vi "Read-Write File Paths setup.vi"(8 "error in":errorcluster, 11 "Function":T1) -> (0 "error out":errorcluster)   [LabVIEW 2020]
uses:
  Typedefs/Read Write Enum.ctl
  Typedefs/Which path.ctl
  Typedefs/File or Folder path or name.ctl
  Calibration/Globals/gl_Calibration globals.vi
  <vilib>/Utility/config.llb/Read Key (String).vi
  <vilib>/Utility/config.llb/NI_LVConfig.lvlib
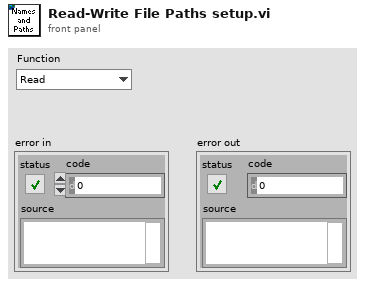
[diagram p1: front panel]
types:
  T1 = typedef "Read Write Enum.ctl" = enum16{"Read", "Write"}
  T2 = typedef "Which path.ctl" = enum16{"Configuration Files", "Calibration Files", "Images", "Setup.ini", "Loaded User profile.ini", "User's-Previous session.ini", "New user profile.ini", "Selected User profile.ini", "User profiles folder", "Power meter scaling.txt", "FOV Cal.ini", "Calibration.ini"}
  T3 = typedef "File or Folder path or name.ctl" = enum16{"Folder name", "Folder path", "File name", "File path & name"}
  T4 = typedef "NI_LVConfig.lvlib/Config Data RefNum.ctl" = refnum<k1>
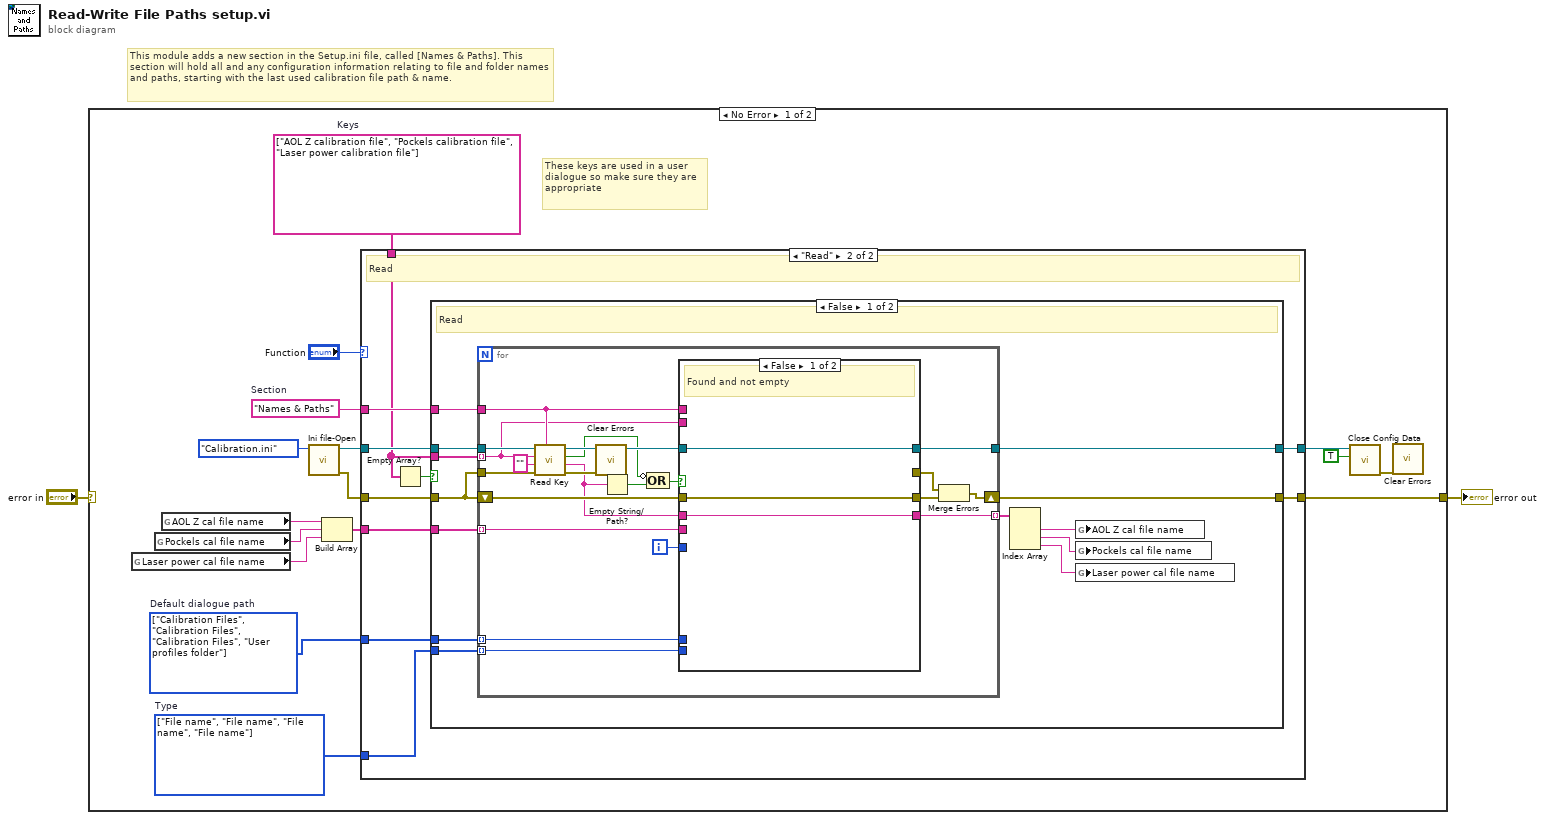
[diagram p0: block diagram]
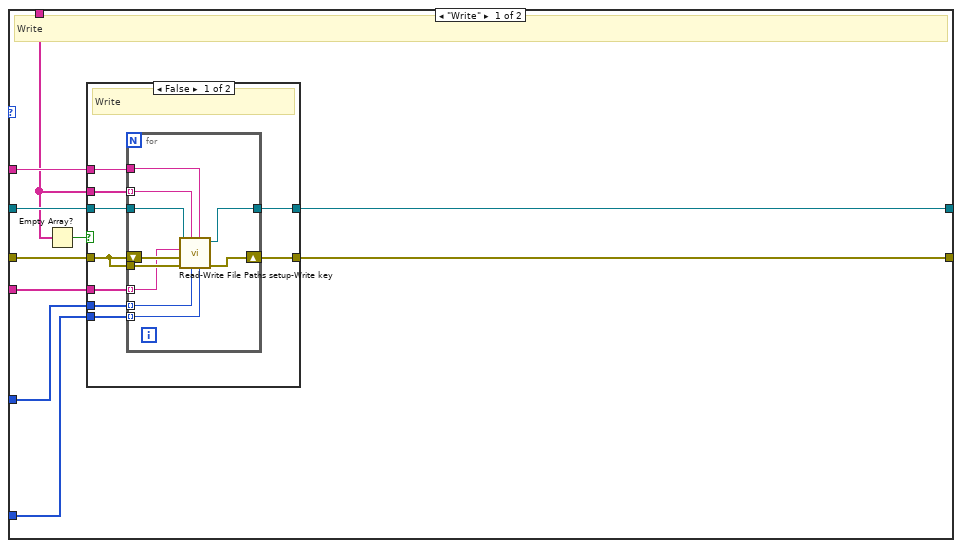
[diagram p2: hidden frame]
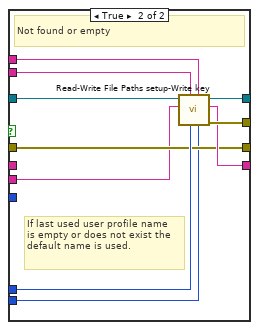
[diagram p4: hidden frame]
diagram:
  # "This module adds a new section in the Setup.ini file, called [Names & Paths]. This section will hold all and any configuration information relating to file and folder names and paths, starting with the last used calibration file path & name."
  n1 = case shown="No Error" "error in" {
    selector: "error in" -> [_ w109]
    tunnel: [w9 w109] -> w2
    frame No Error {
      w6 = T3[] [enum."File name", enum."File name", enum."File name", enum."File name"] items=["Folder name", "Folder path", "File name", "File path & name"]  # Type
      w7 = T2[] [enum."Calibration Files", enum."Calibration Files", enum."Calibration Files", enum."User profiles folder"] items=["Configuration Files", "Calibration Files", "Images", "Setup.ini", "Loaded User profile.ini", "User's-Previous session.ini", "New user profile.ini", "Selected User profile.ini", "User profiles folder", "Power meter scaling.txt", "FOV Cal.ini", "Calibration.ini"]  # Default dialogue path
      w11 = string[] ["AOL Z calibration file", "Pockels calibration file", "Laser power calibration file"]  # Keys
      w18 = "Names & Paths"  # Section
      # "These keys are used in a user dialogue so make sure they are appropriate"
      n2 = global read "gl_Calibration globals.vi" "Laser power cal file name"() -> (w3:string)
      n3 = global read "gl_Calibration globals.vi" "Pockels cal file name"() -> (w4:string)
      n4 = global read "gl_Calibration globals.vi" "AOL Z cal file name"() -> (w5:string)
      n5 = call "Ini file-Open.vi"("Which file?"=Which_path."Calibration.ini") -> ("error out"=w14:errorcluster, "User profile ini file ref"=w15:T4)  [unwired: 7 in, 2 out]
      n6 = Build Array(w5, w4, w3) -> (w10:string[])
      n7 = case shown="\"Read\"" "Function" {
        tunnel: [w28 w58] -> w9
        tunnel: [w27 w59] -> w13
        tunnel: w11 -> [w24 w52]
        tunnel: w14 -> [w22 w54]
        tunnel: w15 -> [w26 w57]
        tunnel: w18 -> [w25 w56]
        tunnel: w10 -> [w21 w53]
        tunnel: w7 -> [w20 w51]
        tunnel: w6 -> [w19 w50]
        frame "Write" {
          # "Write"
          n8 = Empty Array?(array=w24) -> (empty?=w23:bool)
          n9 = case shown="False" w23 {
            tunnel: [w37 w48] -> w28
            tunnel: [w36 w49] -> w27
            tunnel: w24 -> [w35 _]
            tunnel: w26 -> [w34 w49]
            tunnel: w22 -> [w33 w48]
            tunnel: w25 -> [w32 _]
            tunnel: w21 -> [w31 _]
            tunnel: w20 -> [w30 _]
            tunnel: w19 -> [w29 _]
            frame False {
              # "Write"
              n10 = for {
                tunnel: w32 -> [w47]
                tunnel: w34 -> [w46]
                tunnel: w33 -> [w45]
                tunnel: [w44] -> w36
                shift-right: [w43] -> w37
                shift-left: w33 -> [w42]
                tunnel: w35 -> [w40] mode=indexing
                tunnel: w31 -> [w41] mode=indexing
                tunnel: w30 -> [w39] mode=indexing
                tunnel: w29 -> [w38] mode=indexing
                n11 = call "Read-Write File Paths setup-Write key.vi"("Type"=w38, "Section"=w47, "Which file or folder?"=w39, "Key"=w40, "error in (no error)"=w45, "error in"=w42, "Value in"=w41, "Refnum in"=w46) -> ("error out"=w43:errorcluster, "Refnum out"=w44:T4)  [unwired: 1 in, 1 out]
              }
            }
            frame True {
            }
          }
        }
        frame "Read" {
          # "Read"
          n12 = Empty Array?(array=w52) -> (empty?=w55:bool)
          n13 = case shown="False" w55 {
            tunnel: [w71 w108] -> w59
            tunnel: [w70 w107] -> w58
            tunnel: w52 -> [w69 _]
            tunnel: w57 -> [w68 w108]
            tunnel: w54 -> [w67 w107]
            tunnel: w56 -> [w66 _]
            tunnel: w53 -> [w65 _]
            tunnel: w51 -> [w64 _]
            tunnel: w50 -> [w63 _]
            frame False {
              # "Read"
              n14 = for {
                tunnel: w66 -> [w85]
                tunnel: w68 -> [w93]
                tunnel: w67 -> [w92]
                tunnel: [w88] -> w71
                shift-right: [w91] -> w70
                shift-left: w67 -> [w80]
                tunnel: w69 -> [w84] mode=indexing
                tunnel: [w82] -> w72 mode=indexing
                tunnel: w65 -> [w83] mode=indexing
                tunnel: w64 -> [w81] mode=indexing
                tunnel: w63 -> [w74] mode=indexing
                i -> [w73]
                n15 = call-poly <vilib>:"Read Key.vi"("section"=w85, "error in (no error)"=w92, "default value"="" ("Index of E-Stop DI to bypass if DO is TRUE"), "key"=w84, "refnum"=w93) -> ("error out"=w87:errorcluster, "value"=w78:string, "found?"=w76:bool, "refnum out"=w89:T4)  [unwired: 3 in]
                n16 = call <vilib>:"Clear Errors.vi"("error in (no error)"=w87) -> ()  [unwired: 5 in, 2 out]
                n17 = Empty String/Path?(string/path=w78) -> (empty?=w77:bool)
                n18 = Compound Arithmetic op=OR(invert w76, w77) -> (w75:bool)
                n19 = case shown="False" w75 {
                  tunnel: w89 -> [w96 w106]
                  tunnel: [w96 w105] -> w88
                  tunnel: [_ w104] -> w86
                  tunnel: w85 -> [_ w103]
                  tunnel: w84 -> [_ w102]
                  tunnel: w83 -> [_ w97]
                  tunnel: w78 -> [w95 _]
                  tunnel: [w95 w100] -> w82
                  tunnel: w81 -> [_ w101]
                  tunnel: w80 -> [w94 w99]
                  tunnel: [w94 w99] -> w79
                  tunnel: w74 -> [_ w98]
                  tunnel: w73 -> [_ _]
                  frame False {
                    # "Found and not empty"
                  }
                  frame True {
                    # "If last used user profile name \nis empty or does not exist the default name is used."
                    # "Not found or empty"
                    n20 = call "Read-Write File Paths setup-Write key.vi"("Type"=w98, "Section"=w103, "Which file or folder?"=w101, "Key"=w102, "Value in"=w97, "Refnum in"=w106) -> ("error out"=w104:errorcluster, "Value out"=w100:string, "Refnum out"=w105:T4)  [unwired: 3 in]
                  }
                }
                n21 = Merge Errors(w86, w79) -> (w91:errorcluster)
              }
              n22 = Index Array(array=w72) -> (element #1=w62:string, element #2=w61:string, element #3=w60:string)  [unwired: 3 in]
              n23 = global write "gl_Calibration globals.vi" "AOL Z cal file name"(w62) -> ()
              n24 = global write "gl_Calibration globals.vi" "Pockels cal file name"(w61) -> ()
              n25 = global write "gl_Calibration globals.vi" "Laser power cal file name"(w60) -> ()
            }
            frame True {
            }
          }
        }
      }
      n26 = call <vilib>:"Close Config Data.vi"("write file if changed (T)"=TRUE ("write configuration file? (F)"), "refnum"=w13) -> ("error out"=w12:errorcluster)  [unwired: 8 in, 1 out]
      n27 = call <vilib>:"Clear Errors.vi"("error in (no error)"=w12) -> ()  [unwired: 5 in, 2 out]
    }
    frame Error {
    }
  }
  "error out" <- w2
